vi "Device Activate.vi"(8 "error in (no error)":errorcluster, 10 "Activate Mode":T1, 11 "IED in":refnum<class "IED.lvclass">) -> (0 "error out":errorcluster, 3 "IED out":refnum<class "IED.lvclass">)   [LabVIEW 2015, in "IED Actor.lvlib" / "IED.lvclass"]
uses:
  IED.lvclass
  Controls/Device Activate Mode Select.ctl
  <vilib>/ActorFramework/Actor/Actor.lvclass/Actor.ctl
  IED.lvclass/IED.ctl
  SCADA Core/SCADA Abstract Messages/Simple Command Status Msg/Simple Command Status.ctl
  SCADA Core/SCADA Response Messages/Return Activate Status Msg/Return Activate Status Msg.lvclass/Return Activate Status Msg.ctl
  <vilib>/ActorFramework/Message Enqueuer/Message Enqueuer.lvclass/Message Enqueuer.ctl
  SCADA Core/SCADA Abstract Messages/Black Start Status Msg/Black Start Status.ctl
  SCADA Core/SCADA Messages/Return Black Start Status Msg/Return Black Start Status Msg.lvclass/Return Black Start Status Msg.ctl
  SCADA Core/SCADA Abstract Messages/Device Action Status Msg/Device Action Status.ctl
  SCADA Core/SCADA Response Messages/Return Device Activate Status Msg/Return Device Activate Status Msg.lvclass/Return Device Activate Status Msg.ctl
  <vilib>/ActorFramework/Message Enqueuer/Enqueue.vi
  <vilib>/ActorFramework/Message Priority Queue/Priority Enqueue.vi
  SCADA Core/SCADA Response Messages/Return Activate Status Msg/Return Activate Status Msg.lvclass
  SCADA Core/SCADA Messages/Return Black Start Status Msg/Return Black Start Status Msg.lvclass
  SCADA Core/SCADA Response Messages/Return Device Activate Status Msg/Return Device Activate Status Msg.lvclass
  <vilib>/Modbus/master/Modbus Master.lvclass
  <vilib>/ActorFramework/Actor/Actor.lvclass
  SCADA Core/SCADA Abstract Messages/Simple Command Status Msg/Simple Command Status Msg.lvclass
  SCADA Core/SCADA Abstract Messages/Device Action Status Msg/Device Action Status Msg.lvclass
  SCADA Core/SCADA Abstract Messages/Black Start Status Msg/Black Start Status Msg.lvclass
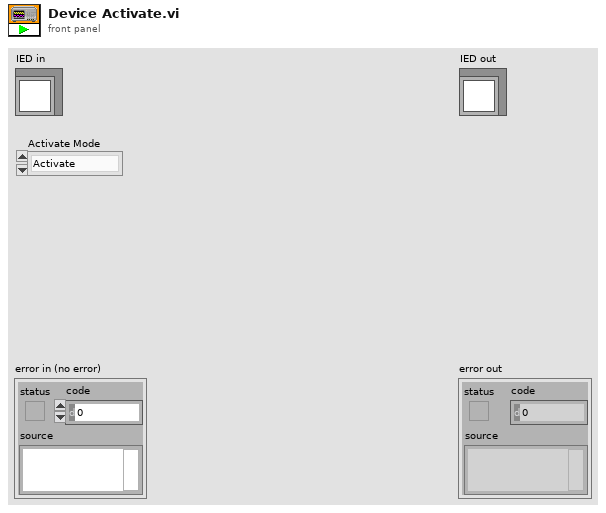
[diagram p1: front panel]
types:
  T1 = typedef "IED Actor.lvlib/IED.lvclass/Device Activate Mode Select.ctl" = enum16{"Activate", "Blackstart", "Individual"}
  T2 = typedef "SCADA Core.lvlib/Simple Command Status Msg.lvclass/Simple Command Status.ctl" = enum16{"Success", "Failure"}
  T3 = typedef "SCADA Core.lvlib/Black Start Status Msg.lvclass/Black Start Status.ctl" = enum16{"Success", "Failure"}
  T4 = typedef "SCADA Core.lvlib/Device Action Status Msg.lvclass/Device Action Status.ctl" = enum16{"Success", "Failure"}
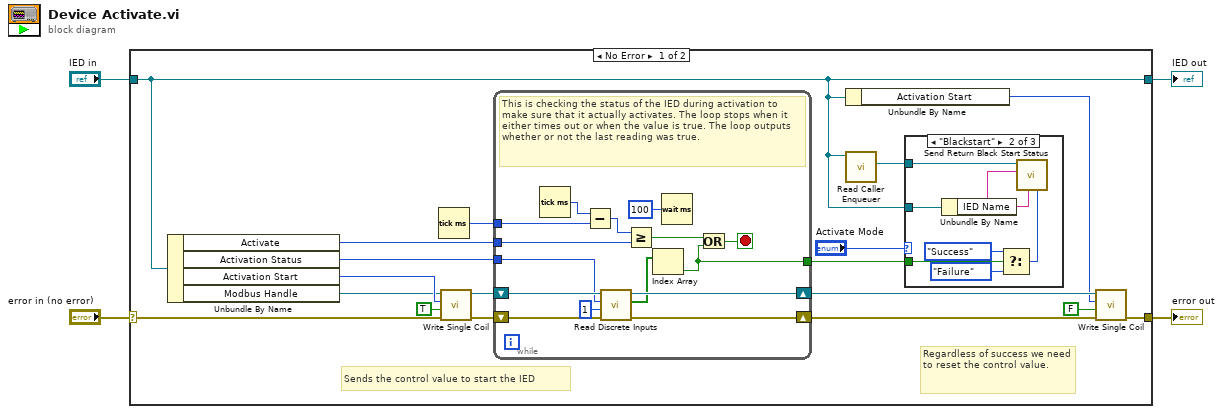
[diagram p0: block diagram]
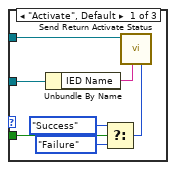
[diagram p2: hidden frame]
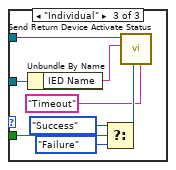
[diagram p3: hidden frame]
diagram:
  n1 = case shown="No Error" "error in (no error)" {
    selector: "error in (no error)" -> [w8 w61]
    tunnel: [w6 w61] -> w3
    tunnel: [w5 w60] -> w1
    tunnel: "IED in" -> [w5 w60]
    frame No Error {
      # "Regardless of success we need to reset the control value."
      # "Sends the control value to start the IED"
      n2 = Unbundle By Name(w5) -> ("Activate"=w16:u32, "Activation Status"=w17:u16, "Activation Start"=w21:u16, "Modbus Handle"=w7:refnum<class "Modbus Master.lvclass">)
      n3 = Tick Count (ms)() -> (millisecond timer value=w22:u32)
      n4 = call-dynamic "Write Single Coil.vi"("error in (no error)"=w8, "coil value"=TRUE, "address"=w21, "Modbus master in"=w7) -> ("error out"=w18:errorcluster, "Modbus master out"=w19:refnum<class "Modbus Master.lvclass">)  [unwired: 6 in]
      n5 = while {
        tunnel: w22 -> [w57]
        tunnel: w16 -> [w55]
        tunnel: w17 -> [w51]
        shift-right: [w45] -> w15
        shift-left: w18 -> [w50]
        tunnel: [w46] -> w10
        shift-right: [w48] -> w14
        shift-left: w19 -> [w52]
        stop <- w53 stop-if-true
        # "This is checking the status of the IED during activation to make sure that it actually activates. The loop stops when it either times out or when the value is true. The loop outputs whether or not the last reading was true."
        n6 = Tick Count (ms)() -> (millisecond timer value=w58:u32)
        n7 = Subtract(x=w58, y=w57) -> (x-y=w56:u32)
        n8 = call-dynamic "Read Discrete Inputs.vi"("error in (no error)"=w50, "number of discrete inputs"=u16 1 ("number of coils"), "starting address"=w51, "Modbus master in"=w52) -> ("error out"=w45:errorcluster, "discrete input values"=w47:bool[], "Modbus master out"=w48:refnum<class "Modbus Master.lvclass">)  [unwired: 5 in]
        n9 = Greater Or Equal?(x=w56, y=w55) -> (x >= y?=w54:bool)
        n10 = Index Array(array=w47) -> (element=w46:bool)  [unwired: 1 in]
        n11 = Wait (ms)(milliseconds to wait=u32 100) -> ()  [unwired: 1 out]
        n12 = Or(x=w54, y=w46) -> (x .or. y?=w53:bool)
      }
      n13 = Unbundle By Name(w5) -> ("Activation Start"=w13:u16)
      n14 = call <vilib>:"Read Caller Enqueuer.vi"("Actor"=w5) -> ("Caller Enqueuer"=w11:refnum<class "Message Enqueuer.lvclass">)  [unwired: 10 in]
      n15 = case shown="\"Blackstart\"" "Activate Mode" {
        tunnel: w11 -> [w29 w34 w44]
        tunnel: w10 -> [w28 w36 w43]
        tunnel: w5 -> [w23 w35 w39]
        frame "Activate", Default {
          n16 = Unbundle By Name(w23) -> ("IED Name"=w25:string)
          n17 = Select(t=Simple_Command_Status."Success" ("Status"), s=w28, f=Simple_Command_Status."Failure" ("Status")) -> (s? t:f=w24:T2)
          n18 = call "Send Return Activate Status.vi"("Status"=w24, "error"=w25, "Message Enqueuer"=w29) -> ()  [unwired: 7 in, 2 out]
        }
        frame "Blackstart" {
          n19 = Unbundle By Name(w35) -> ("IED Name"=w33:string)
          n20 = Select(t=Black_Start_Status."Success" ("Status"), s=w36, f=Black_Start_Status."Failure" ("Status")) -> (s? t:f=w30:T3)
          n21 = call "Send Return Black Start Status.vi"("Status"=w30, "error"=w33, "IED Name"=w33, "Message Enqueuer"=w34) -> ()  [unwired: 6 in, 2 out]
        }
        frame "Individual" {
          n22 = Unbundle By Name(w39) -> ("IED Name"=w38:string)
          n23 = Select(t=Device_Action_Status."Success" ("Status"), s=w43, f=Device_Action_Status."Failure" ("Status")) -> (s? t:f=w40:T4)
          n24 = call "Send Return Device Activate Status.vi"("error string"="Timeout", "Status"=w40, "IED Name"=w38, "Message Enqueuer"=w44) -> ()  [unwired: 6 in, 2 out]
        }
      }
      n25 = call-dynamic "Write Single Coil.vi"("error in (no error)"=w15, "coil value"=FALSE, "address"=w13, "Modbus master in"=w14) -> ("error out"=w6:errorcluster)  [unwired: 6 in, 1 out]
    }
    frame Error {
    }
  }
  "error out" <- w3
  "IED out" <- w1
